vi "VNA_Set_PowerLevel.vi"(2 "error in (no error)":errorcluster, 3 "Level":dbl, 4 "VISA in":refnum<visa-resource-name>) -> (0 "error out":errorcluster, 1 "VISA out":refnum<visa-resource-name>)   [LabVIEW 2017]
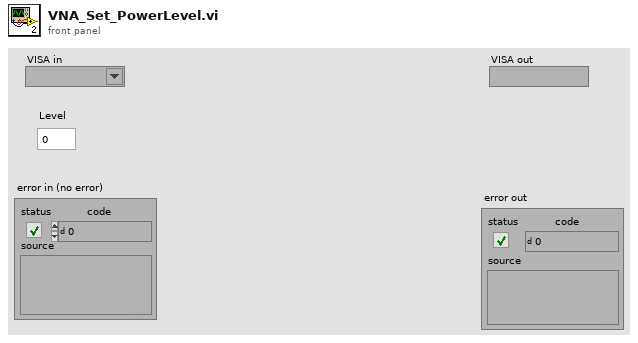
[diagram p1: front panel]
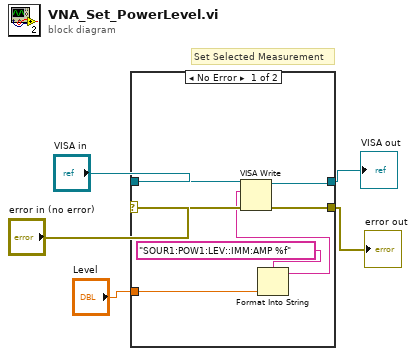
[diagram p0: block diagram]
diagram:
  # "Set Selected Measurement"
  n1 = case shown="No Error" "error in (no error)" {
    selector: "error in (no error)" -> [w12 w14]
    tunnel: [w9 w14] -> w3
    tunnel: "VISA in" -> [w11 w13]
    tunnel: [w10 w13] -> w2
    tunnel: "Level" -> [w6 _]
    frame No Error {
      n2 = Format Into String(format string="SOUR1:POW1:LEV::IMM:AMP %f" ("Cmdline"), w6) -> (resulting string=w7:string)  [unwired: 2 in, 1 out]
      n3 = VISA Write(VISA resource name=w11, write buffer=w7, error in (no error)=w12) -> (VISA resource name out=w10:refnum<visa-resource-name>, error out=w9:errorcluster)  [unwired: 1 out]
    }
    frame Error {
    }
  }
  "error out" <- w3
  "VISA out" <- w2
